vi "Join Doubles with Comma.vi"(1 "double array":dbl[](array[numeric])) -> (0 "joined string":string)   [LabVIEW 2021, in "PMIC Common.lvlib"]
uses:
  PMIC Common.lvlib
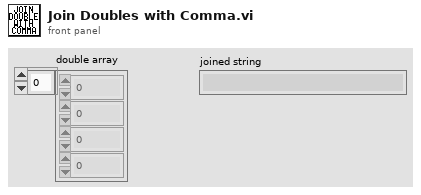
[diagram p1: front panel]
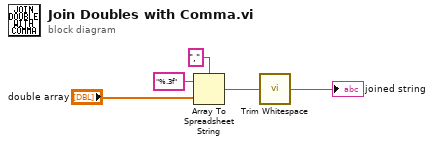
[diagram p0: block diagram]
diagram:
  n1 = Array To Spreadsheet String(delimiter (Tab)=",", array="double array", 3:"%.3f" ("format string")) -> (spreadsheet string=w2:string)
  n2 = call <vilib>:"Trim Whitespace.vi"("string"=w2) -> ("trimmed string"=→"joined string":string)  [unwired: 1 in]
